vi "Get Network Interfaces Info.vi"(8 "Error In":errorcluster, 11 "Install LV Data":T3={"SSH Session"=refnum, "Status Log"="", "Detailed Log"="", "Credentials"={"Hostname or IP"="192.168.7.2", "Username"="root", "Password"=""}, "Target Info"={"OS Version"="", "CPU"="", "Systemd Version"="", "Internet Access"=FALSE, "Device Type"="", "LV Installed Ver"="", "LV Available Ver"="", "LV Upgrade Available"=FALSE, "Hostname"="", "NIC Info"=[]}, "Reboot Required?"=FALSE}) -> (0 "Error Out":errorcluster, 3 "Install LV Data":T3={"SSH Session"=refnum, "Status Log"="", "Detailed Log"="", "Credentials"={"Hostname or IP"="192.168.7.2", "Username"="root", "Password"=""}, "Target Info"={"OS Version"="", "CPU"="", "Systemd Version"="", "Internet Access"=FALSE, "Device Type"="", "LV Installed Ver"="", "LV Available Ver"="", "LV Upgrade Available"=FALSE, "Hostname"="", "NIC Info"=[]}, "Reboot Required?"=FALSE})   [LabVIEW 2020, in "LMH-LINX.lvlib"]
uses:
  LMH-LINX.lvlib
  Install LV Data.ctl
  Target Info.ctl
  NIC Info.ctl
  NIC Mode.ctl
panel:
  out "Target Info.NIC Info":T1[](array[typedef])
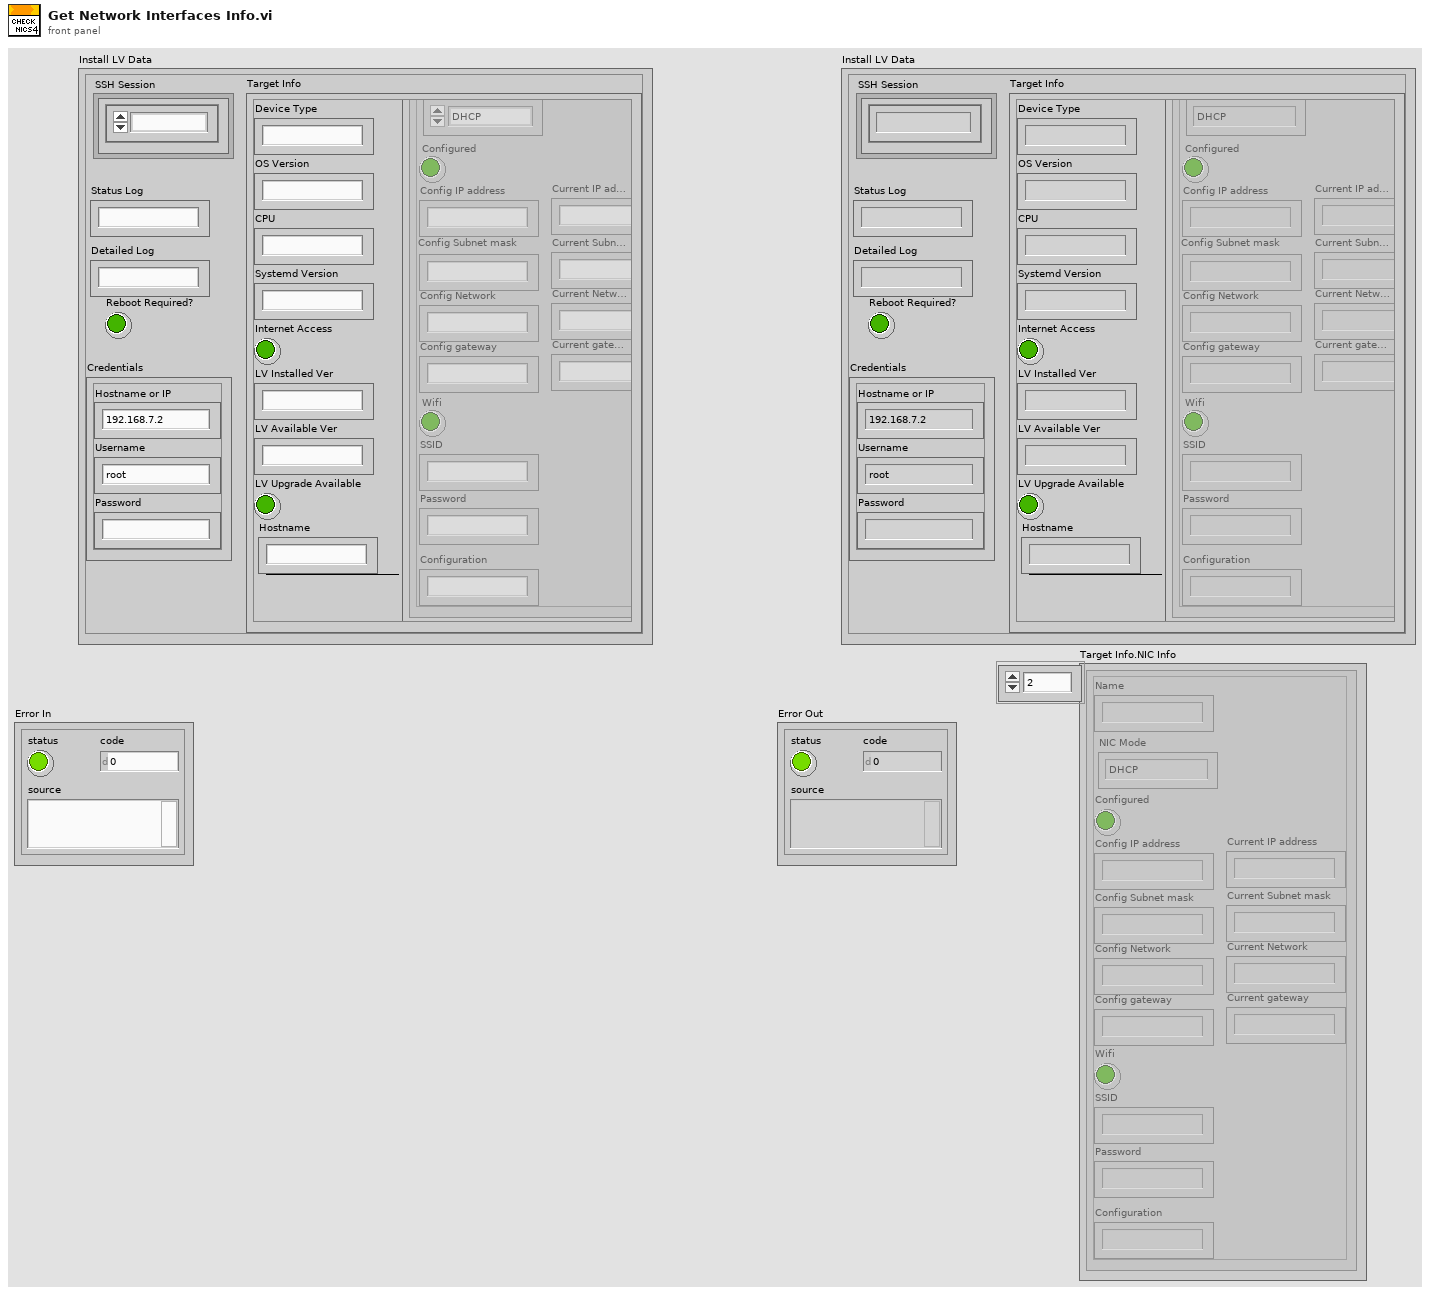
[diagram p1: front panel]
types:
  T1 = typedef "LMH-LINX.lvlib/NIC Info.ctl" = cluster{"Name":string, "NIC Mode":T2, "Configured":bool, "Config IP address":string, "Config Subnet mask":string, "Config Network":string, "Config gateway":string, "Wifi":bool, "SSID":string, "Password":string, "Configuration":string, "Current IP address":string, "Current Subnet mask":string, "Current gateway":string, "Current Network":string}
  T2 = typedef "LMH-LINX.lvlib/NIC Mode.ctl" = enum16{"DHCP", "Static", "Loopback"}
  T3 = typedef "LMH-LINX.lvlib/Install LV Data.ctl" = cluster{"SSH Session":refnum<k1>, "Status Log":string, "Detailed Log":string, "Credentials":cluster{"Hostname or IP":string, "Username":string, "Password":string}, "Target Info":T4, "Reboot Required?":bool}
  T4 = typedef "LMH-LINX.lvlib/Target Info.ctl" = cluster{"OS Version":string, "CPU":string, "Systemd Version":string, "Internet Access":bool, "Device Type":string, "LV Installed Ver":string, "LV Available Ver":string, "LV Upgrade Available":bool, "Hostname":string, "NIC Info":T1[]}
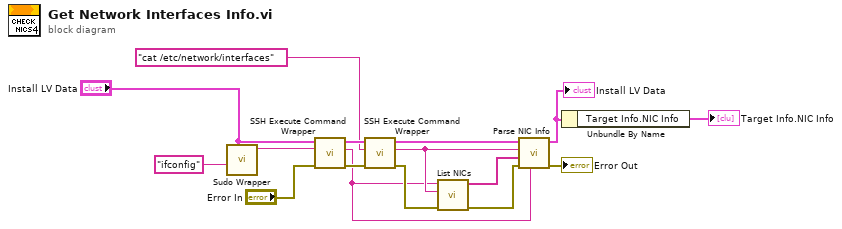
[diagram p0: block diagram]
diagram:
  n1 = call "Sudo Wrapper.vi"("Install LV Data"="Install LV Data", "comand string"="ifconfig" ("Command")) -> ("combined command string"=w2:string)  [unwired: 9 in]
  n2 = call "SSH Execute Command Wrapper.vi"("Error In"="Error In", "Command"=w2, "Install LV Data in"="Install LV Data") -> ("Error Out"=w6:errorcluster, "Std Out"=w4:string, "Install LV Data out"=w12:T3)  [unwired: 6 in]
  n3 = call "SSH Execute Command Wrapper.vi"("Error In"=w6, "Command"="cat /etc/network/interfaces", "Install LV Data in"=w12) -> ("Error Out"=w7:errorcluster, "Std Out"=w9:string, "Install LV Data out"=w11:T3)  [unwired: 6 in]
  n4 = call "List NICs.vi"("Error In"=w7, "Network Interface Config"=w9, "ifconfig"=w4) -> ("Error Out"=w5:errorcluster, "All NICs"=w15:string[])  [unwired: 7 in]
  n5 = call "Parse NIC Info.vi"("ifconfig"=w4, "Error In"=w5, "All NICs"=w15, "interfaces config"=w9, "Install LV Data"=w11) -> ("Error Out"=→"Error Out":errorcluster, "Install LV Data"=w8:T3)  [unwired: 5 in]
  "Install LV Data" <- w8
  n6 = Unbundle By Name(w8) -> ("Target Info.NIC Info"=→"Target Info.NIC Info":T1[])
